vi "Rename.vi"(8 "error in (no error)":errorcluster, 9 "New name":string, 10 "ProjectItem Refnum":refnum<vi>, 11 "PPL in":refnum<class "NI_AB_API_DPPL.lvclass">) -> (0 "error out":errorcluster, 3 "PPL out":refnum<class "NI_AB_API_DPPL.lvclass">)   [LabVIEW 2020, in "NI_AB_API_DPPL.lvclass"]
uses:
  <vilib>/AppBuilder/AB_API/DPPL/NI_AB_API_DPPL.lvclass
  <vilib>/AppBuilder/AB_API/PPL/NI_AB_API_PPL.lvclass
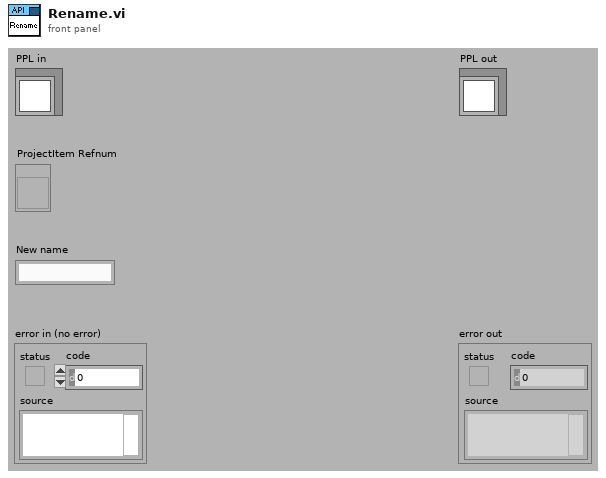
[diagram p1: front panel]
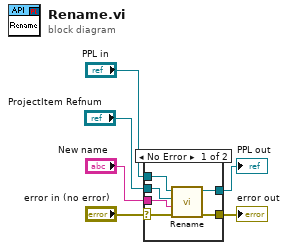
[diagram p0: block diagram]
diagram:
  n1 = case shown="No Error" "error in (no error)" {
    selector: "error in (no error)" -> [w9 w14]
    tunnel: [w10 w14] -> w5
    tunnel: [w11 w13] -> w3
    tunnel: "PPL in" -> [w12 w13]
    tunnel: "New name" -> [w7 _]
    tunnel: "ProjectItem Refnum" -> [w8 _]
    frame No Error {
      n2 = call-parent "Rename.vi"("error in (no error)"=w9, "New name"=w7, "ProjectItem Refnum"=w8, "PPL in"=w12) -> ("error out"=w10:errorcluster, "PPL out"=w11:refnum<class "NI_AB_API_DPPL.lvclass">)  [unwired: 6 in]
    }
    frame Error {
    }
  }
  "error out" <- w5
  "PPL out" <- w3
